vi "Get Loop Time.vi"() -> (0 "Loop Time":u32(graph))   [LabVIEW 2012]
panel:
  out "Min Loop Time":u32
  out "Max Loop Time":u32
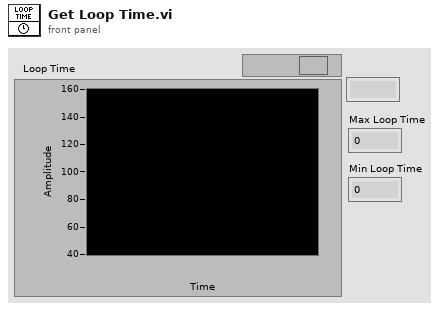
[diagram p1: front panel]
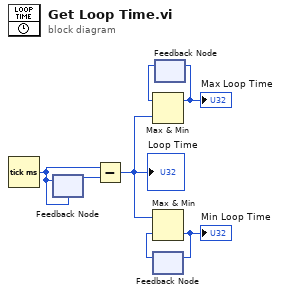
[diagram p0: block diagram]
diagram:
  n1 = Tick Count (ms)() -> (millisecond timer value=w6:u32)
  n2 = feedback #1(w6) -> (w7:u32)
  n3 = feedback-in #1(w6) -> ()
  n4 = Subtract(x=w6, y=w7) -> (x-y=w3:u32)
  "Loop Time" <- w3
  n5 = feedback #2() -> (w2:u32)  [unwired: 1 in]
  n6 = Max & Min(x=w3, y=w2) -> (min(x,y)=w1:u32)  [unwired: 1 out]
  "Min Loop Time" <- w1
  n7 = feedback-in #2(w1) -> ()
  n8 = feedback #3() -> (w4:u32)  [unwired: 1 in]
  n9 = Max & Min(x=w4, y=w3) -> (max(x,y)=w5:u32)  [unwired: 1 out]
  "Max Loop Time" <- w5
  n10 = feedback-in #3(w5) -> ()
